vi "Space.vi"() -> (3 "_":u8)   [LabVIEW 2021, in "d22.lvlib"]
uses:
  d22.lvlib
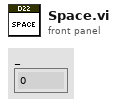
[diagram p1: front panel]
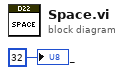
[diagram p0: block diagram]
diagram:
  "_" <- u8 32 ("element")
